vi "other.vi"() -> ()   [LabVIEW 2011]
uses:
  <vilib>/DAQmx/write.llb/DAQmx Write (Analog DBL 1Chan 1Samp).vi
  <vilib>/DAQmx/miscellaneous.llb/DAQmx Fill In Error Info.vi
  <vilib>/NI_Real-Time Target Support.lvlib
  <vilib>/measure/NI_MABase.lvlib
panel:
  out "Numeric":dbl
  in  "amplitude":dbl=1.0 format="%0.2p"
  in  "frequency":dbl=10.0 format="%0.2p"
  in  "signal type":T1(ring)
  out "PXI6281Task":refnum<k21>
  in  "stop":bool
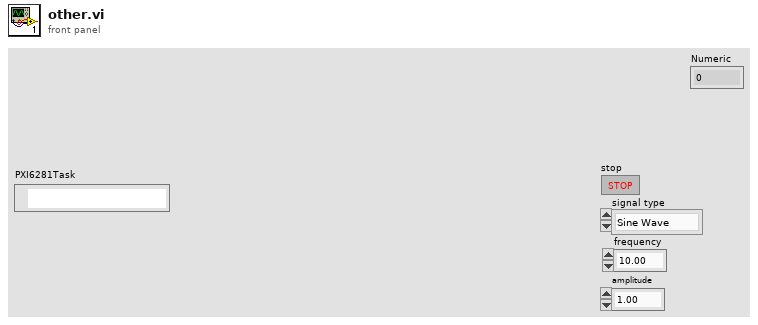
[diagram p1: front panel]
types:
  T1 = enum16{"Sine Wave", "Triangle Wave", "Square Wave", "Sawtooth Wave"}
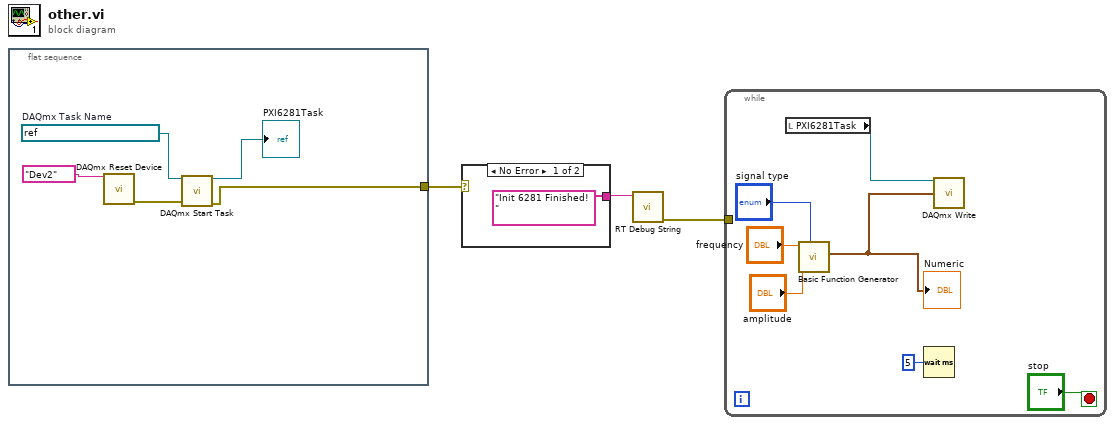
[diagram p0: block diagram]
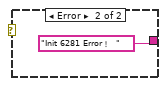
[diagram p2: hidden frame]
diagram:
  n1 = flat-sequence {
    tunnel: [w4] -> w2
    frame #0 {
      w7 = refnum<k21> "ProjectVoltageOutTask"  # DAQmx Task Name
      n2 = call <vilib>:"DAQmx Reset Device.vi"("device in"=tag "Dev2") -> ("error out"=w6:errorcluster)  [unwired: 14 in]
      n3 = call <vilib>:"DAQmx Start Task.vi"("task/channels in"=w7, "error in"=w6) -> ("task out"=→"PXI6281Task":refnum<k21>, "error out"=w4:errorcluster)  [unwired: 12 in]
    }
  }
  n4 = case shown="No Error" w2 {
    tunnel: ["Init 6281 Finished!   " ("String to write") "Init 6281 Error！  " ("String to write")] -> w3
    frame No Error {
    }
    frame Error {
    }
  }
  n5 = call <vilib>:"RT Debug String.vi"("String to write"=w3) -> ("error out"=w1:errorcluster)  [unwired: 10 in]
  n6 = while {
    tunnel: w1 -> [_]
    stop <- "stop" stop-if-true
    n7 = local read "PXI6281Task"() -> (w15:refnum<k21>)
    n8 = call <vilib>:"Basic Function Generator.vi"("signal type"="signal type", "amplitude"="amplitude", "frequency"="frequency") -> ("signal out"=w11:waveform(dbl))  [unwired: 6 in, 2 out]
    "Numeric" <- w11
    n9 = Wait (ms)(milliseconds to wait=u32 5) -> ()  [unwired: 1 out]
    n10 = call-poly <vilib>:"DAQmx Write.vi"("task/channels in"=w15, "data"=w11) -> ()  [unwired: 11 in, 3 out]
  }
